vi "debug.vi"() -> ()   [LabVIEW 2013]
uses:
  source/Serializer.PlainText/Serializer.PlainText.lvclass
  source/Serializer/Serializer.lvclass
panel:
  out "data":cluster{"String":string, "Array":dbl[]}[](array[cluster])
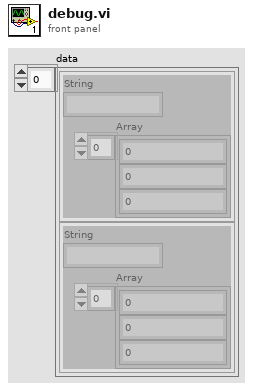
[diagram p1: front panel]
types:
  T1 = cluster{"String":string, "Cluster Array":cluster{"String":string, "Number":dbl}[]}
  T2 = cluster{"String":string, "Cluster 2":cluster{"String":string, "Number":dbl}}
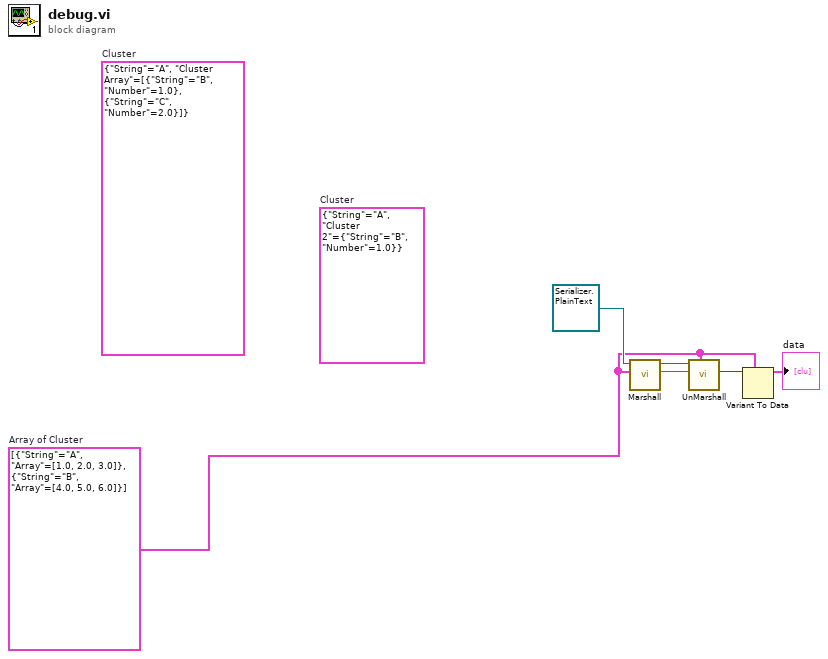
[diagram p0: block diagram]
diagram:
  w2 = cluster{"String":string, "Array":dbl[]}[] [{"String"="A", "Array"=[1.0, 2.0, 3.0]}, {"String"="B", "Array"=[4.0, 5.0, 6.0]}]  # Array of Cluster
  (unwired) T1 {"String"="A", "Cluster Array"=[{"String"="B", "Number"=1.0}, {"String"="C", "Number"=2.0}]}  # Cluster
  (unwired) T2 {"String"="A", "Cluster 2"={"String"="B", "Number"=1.0}}  # Cluster
  n1 = call "Marshall.vi"("Variant"=w2, "Serializer in"=refnum<class "Serializer.PlainText.lvclass"> refnum ("Serializer.PlainText.lvclass")) -> ("String"=w4:string, "Serializer out"=w5:refnum<class "Serializer.PlainText.lvclass">)  [unwired: 7 in, 1 out]
  n2 = call "UnMarshall.vi"("Type"=w2, "String"=w4, "Serializer in"=w5) -> ("Variant"=w6:variant)  [unwired: 6 in, 2 out]
  n3 = Variant To Data(type=w2, Variant=w6) -> (data=→"data":cluster{"String":string, "Array":dbl[]}[])  [unwired: 1 in, 1 out]
